vi "Initiate_Motion.vi"(6 "Error In":errorcluster, 8 "Node":i32, 9 "Serial In":refnum<visa-resource-name>) -> (0 "Error Out":errorcluster, 3 "Serial Out":refnum<visa-resource-name>)   [LabVIEW 2019]
uses:
  <vilib>/Utility/error.llb/Error Cluster From Error Code.vi
  <vilib>/ErrorRing/Error Ring.xnode
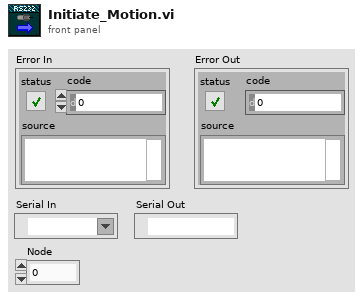
[diagram p1: front panel]
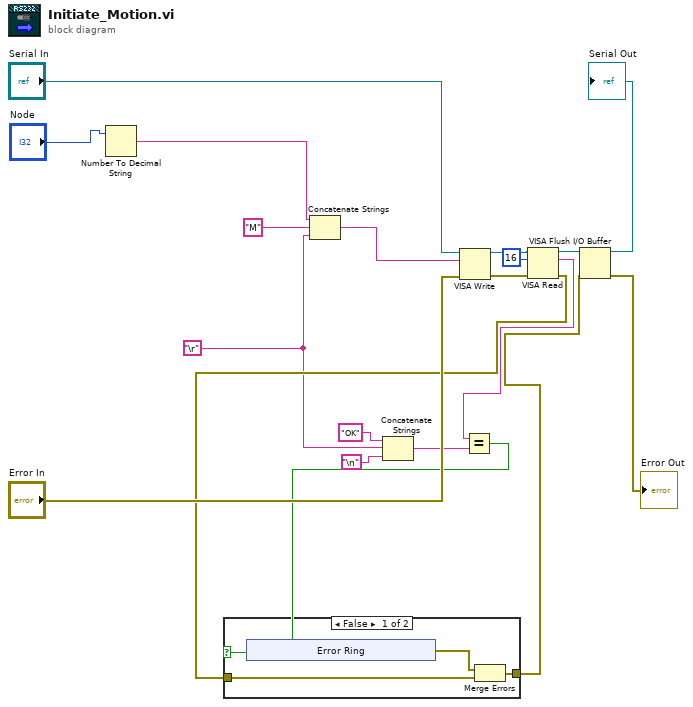
[diagram p0: block diagram]
diagram:
  w3 = "\r"
  n1 = Number To Decimal String(number="Node") -> (decimal integer string=w17:string)  [unwired: 1 in]
  n2 = Concatenate Strings(w17, "M" ("string"), w3) -> (w16:string)
  n3 = Concatenate Strings("OK" ("y"), w3, "\n") -> (w2:string)
  n4 = VISA Write(VISA resource name="Serial In", write buffer=w16, error in (no error)="Error In") -> (VISA resource name out=w10:refnum<visa-resource-name>, error out=w9:errorcluster)  [unwired: 1 out]
  n5 = VISA Read(VISA resource name=w10, byte count=u32 16, error in (no error)=w9) -> (VISA resource name out=w8:refnum<visa-resource-name>, read buffer=w6:string, error out=w7:errorcluster)  [unwired: 1 out]
  n6 = Equal?(x=w6, y=w2) -> (x = y?=w12:bool)
  n7 = case shown="False" w12 {
    tunnel: w7 -> [w22 w29]
    tunnel: [w23 w29] -> w5
    frame False {
      n8 = xnode "Error Ring"() -> ("error out"=w21:errorcluster)
      n9 = Merge Errors(w21, w22) -> (w23:errorcluster)
    }
    frame True {
    }
  }
  n10 = VISA Flush I/O Buffer(VISA resource name=w8, error in (no error)=w5) -> (VISA resource name out=→"Serial Out":refnum<visa-resource-name>, error out=→"Error Out":errorcluster)  [unwired: 1 in]
